vi "Probe.vi"   [LabVIEW 2010]
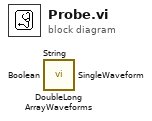
[diagram p0: block diagram]
diagram:
  n1 = call <userlib>:"DoubleLong.vi"() -> ()  [unwired: 11 in, 1 out]
  n2 = call <userlib>:"String.vi"() -> ()  [unwired: 11 in, 1 out]
  n3 = call <userlib>:"Boolean.vi"() -> ()  [unwired: 11 in, 1 out]
  n4 = call <userlib>:"SingleWaveform.vi"() -> ()  [unwired: 11 in, 1 out]
  n5 = call <userlib>:"ArrayWaveforms.vi"() -> ()  [unwired: 11 in, 1 out]
